vi "Display Input (DBL) Popup.vi"(6 "Theme":refnum<class "Theme.lvclass">, 8 "error in":errorcluster, 9 "Default Input":dbl, 10 "Message":string, 11 "Graphic":T1="info") -> (0 "error out":errorcluster, 1 "Input Value":dbl format="%#.10g")   [LabVIEW 2021, in "Pop-Up.lvlib" / "Input (DBL).lvclass"]
doc: "The input (DBL) popup will display information to the user and wait for the operator to enter a value and click the button.\n\n<b>Note:</b> The function <b>Close Pop-Up (DBL).vi</b> can be used to send a value when closing this dialog. Otherwise, use Close Pop-Up.vi to close it early.\n\nInputs:\n-Graphic [typedef combobox] - Image (PNG) for Graphic for Popup\n-Message [String] - String Variable to populate Display\n-Theme [lvclass] - the theme for the style of the popup\n-Default Input [DBL] - default value for the prompt\n\nOutputs\n-Input Value [DBL] - the user's entered data\n\n<b>Code Developed By:</b>\nDaniel Coons\nTechnology Service Corporation\n1983 S Liberty Drive\nBloomington, IN 47403\nPhone: 812 558-7100\ndaniel.coons@tsc.com\nwww.tsc.com/atcs"
uses:
  Input (DBL).lvclass
  Graphics.ctl
  Theme/Theme.lvclass
  Input (DBL).lvclass/Input (DBL).ctl
  Pop-Up.lvlib
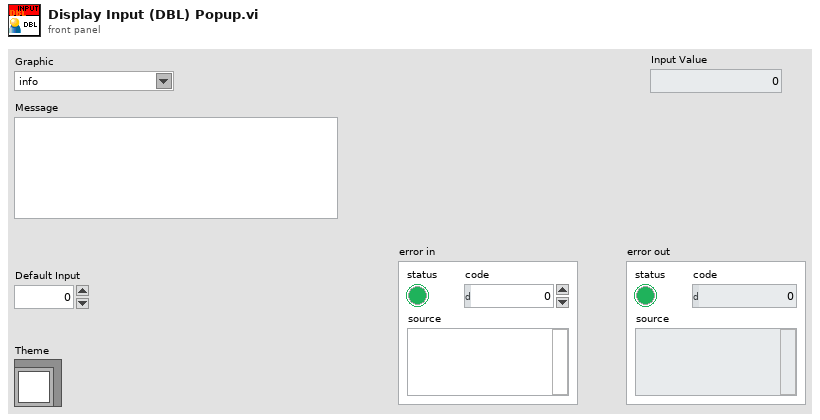
[diagram p1: front panel]
types:
  T1 = typedef "Pop-Up.lvlib/Graphics.ctl" = string
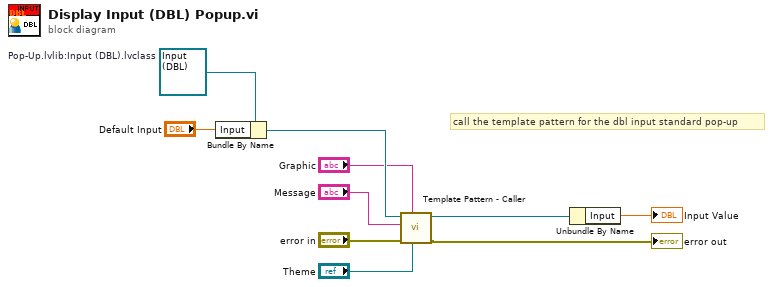
[diagram p0: block diagram]
diagram:
  w8 = refnum<class "Input (DBL).lvclass"> refnum  # Pop-Up.lvlib:Input (DBL).lvclass
  # "call the template pattern for the dbl input standard pop-up"
  n1 = Bundle By Name(cluster=w8, "Input"="Default Input") -> (w6:refnum<class "Input (DBL).lvclass">)
  n2 = call-dynamic "Template Pattern - Caller.vi"("Theme"="Theme", "standard"="Graphic", "error in (no error)"="error in", "Message"="Message", "Pop-Up in"=w6) -> ("error out"=→"error out":errorcluster, "Pop-Up out"=w1:refnum<class "Input (DBL).lvclass">)  [unwired: 5 in]
  n3 = Unbundle By Name(w1) -> ("Input"=→"Input Value":dbl)
